vi "Read_Parameter_From_Data_Packet.vi"(8 "error in (no error)":errorcluster, 11 "Parameter name":string) -> (0 "error out":errorcluster, 3 "Parameter value out":string)   [LabVIEW 2017]
uses:
  Controls/Data Packets/Data_Packet_FGV_Commands.ctl
panel:
  out "Target test parameter value":string
  in  "Target test parameter":string
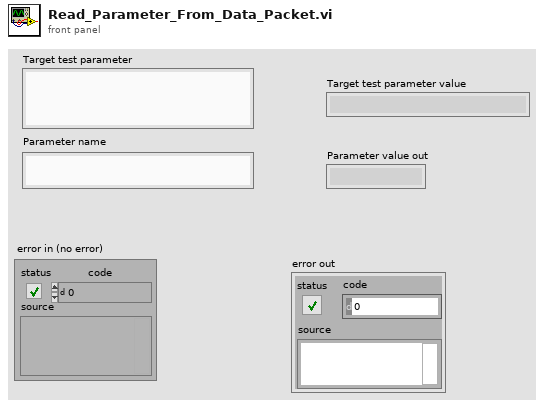
[diagram p1: front panel]
types:
  T1 = typedef "Data_Packet_FGV_Commands.ctl" = enum16{"Update all parameters from data packets", "Update Packet", "Load", "Read Packet Parameters", "Write Packet Parameters", "Read Packet Parameter", "Write Packet Parameter", "Read Data Packets", "Read Data Packet", "Read Data Packet by Parameter Name", "Get Parameter Node and Frame ID", "Read Data Packet from Node ID and Frame ID"}
  T2 = typedef "Data_Packet.ctl" = cluster{"Packet":T3, "Parameters":T7[], "Last Received Time (ms)":u64, "Receive count":i32, "Transmit count":i32, "Transmit interval (ms)":u32, "Last Transmitted Time (ms)":u64, "Receive interval (ms)":u32, "Transmit_Mode":T9, "Transmit Enable":bool, "Cyclic Transmit interval (ms)":u32}
  T3 = typedef "Packet.ctl" = cluster{"Raw Bytes":u8[], "Checksum":bool, "Direction":T4, "Processed Bytes":u8[], "Node ID":u8, "Packet type":T5, "Frame Data":u32, "Priority":T6, "Frame ID":u8}
  T4 = typedef "Packet_Direction.ctl" = enum16{"Transmit", "Receive", "Bidirectional"}
  T5 = typedef "Packet_Type.ctl" = enum16{"Data", "Connection Management", "Remote Request", "Error/Status"}
  T6 = typedef "Packet_Priority.ctl" = enum16{"LOW", "HIGH"}
  T7 = typedef "Parameter.ctl" = cluster{"Parameter name":string, "Node name":string, "Node ID":u8, "Frame name":string, "Frame ID":u8, "Data type":T8, "Start Bit":i32, "Bit Length":i32, "Factor":dbl, "Offset":dbl, "Minimum":dbl, "Maximum":dbl, "Descriptor":string, "Enum values":string[], "Value":string}
  T8 = typedef "Parameter_Data_Type.ctl" = enum16{"BOOL", "UNSIGNED", "SIGNED", "FLOAT32", "ENUM"}
  T9 = typedef "Data_Packet_Transmit_Mode.ctl" = enum16{"Disabled", "Single", "Cyclic"}
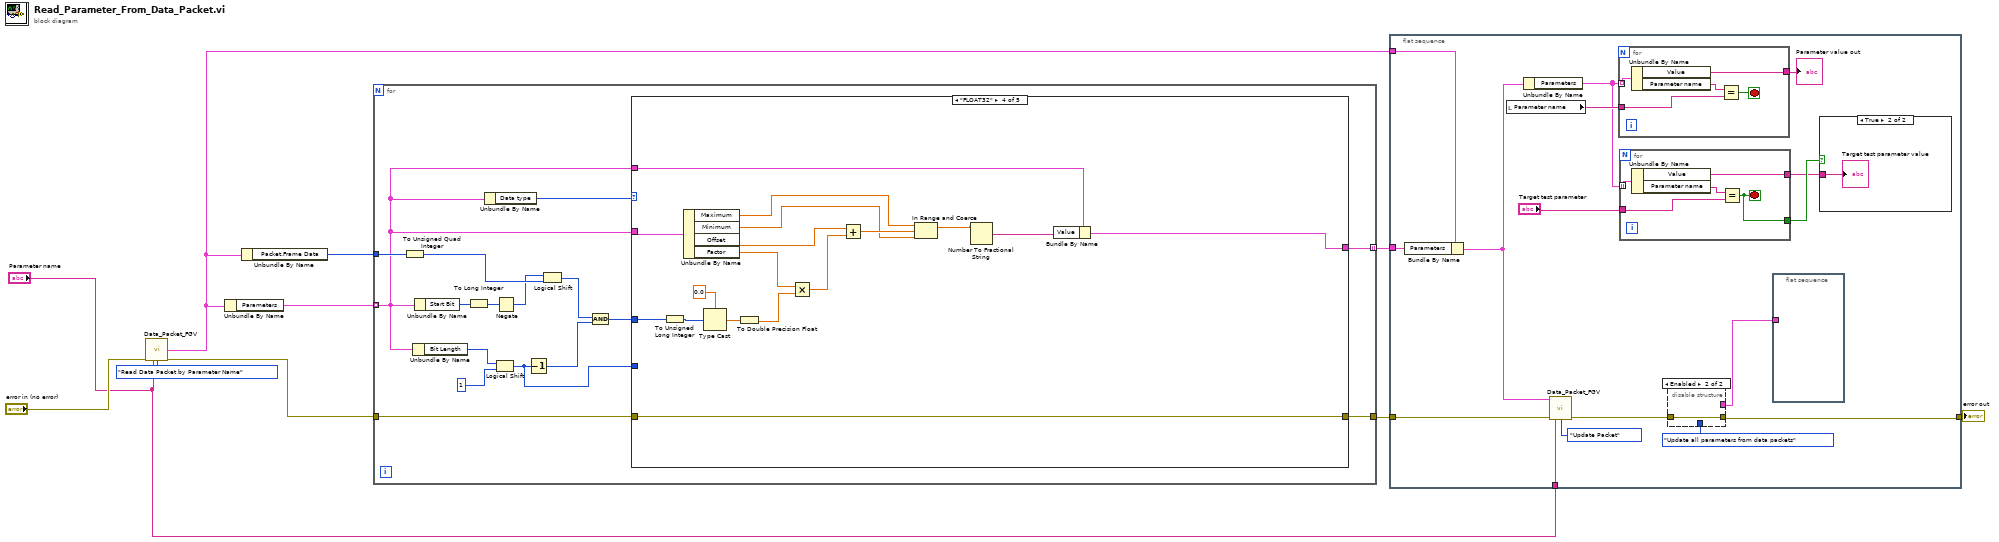
[diagram p0: block diagram]
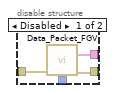
[diagram p2: hidden frame]
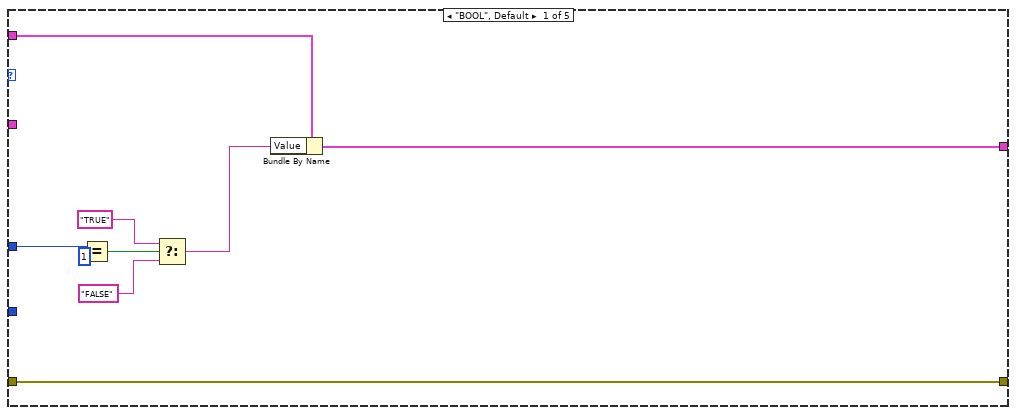
[diagram p4: hidden frame]
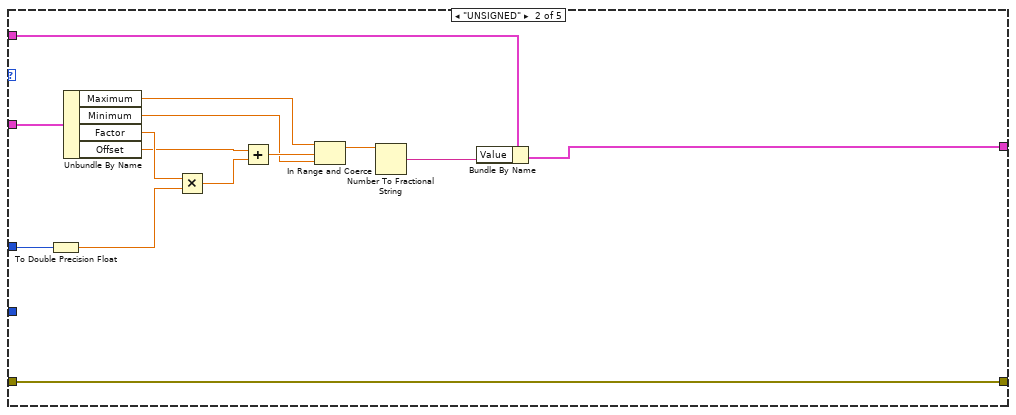
[diagram p5: hidden frame]
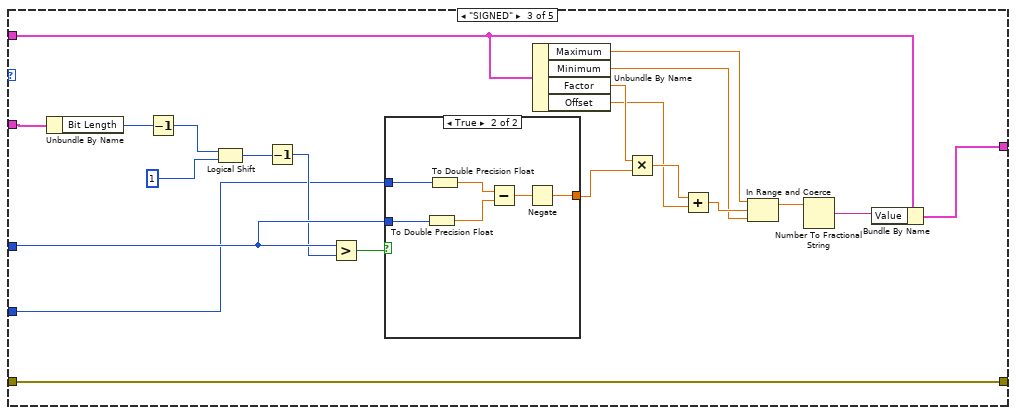
[diagram p6: hidden frame]
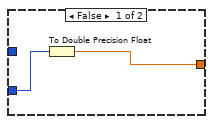
[diagram p7: hidden frame]
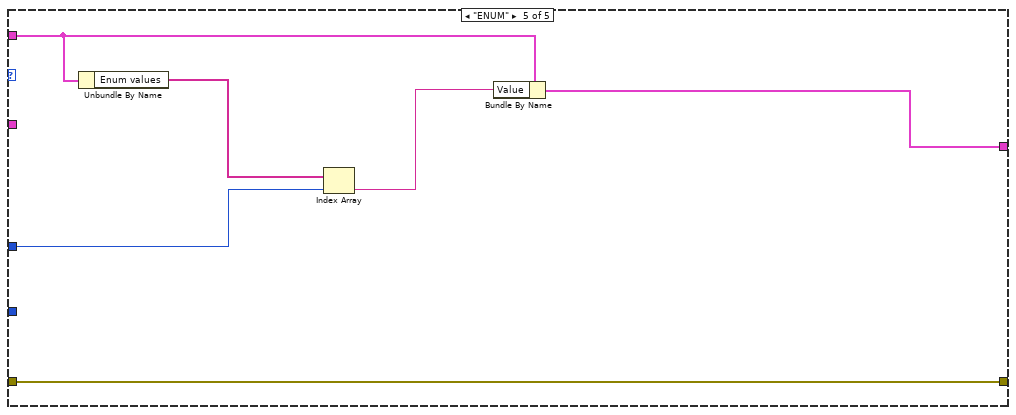
[diagram p8: hidden frame]
diagram:
  n1 = call "Data_Packet_FGV.vi"("error in (no error)"="error in (no error)", "Parameter name"="Parameter name", "Commands"=Data_Packet_FGV_Commands."Read Data Packet by Parameter Name") -> ("Data_Packet out"=w1:T2, "error out"=w7:errorcluster)  [unwired: 7 in, 4 out]
  n2 = Unbundle By Name(w1) -> ("Parameters"=w6:T7[])
  n3 = Unbundle By Name(w1) -> ("Packet.Frame Data"=w8:u32)
  n4 = for {
    tunnel: w8 -> [w26]
    tunnel: w7 -> [w15]
    tunnel: w6 -> [w13] mode=indexing
    tunnel: [w16] -> w3 mode=indexing
    tunnel: [w14] -> w5
    n5 = To Unsigned Quad Integer(1:w26) -> (0:w25:u64)
    n6 = Unbundle By Name(w13) -> ("Bit Length"=w20:i32)
    n7 = Unbundle By Name(w13) -> ("Start Bit"=w24:i32)
    n8 = To Long Integer(number=w24) -> (32bit integer=w23:i32)
    n9 = Unbundle By Name(w13) -> ("Data type"=w18:T8)
    n10 = Logical Shift(y=w20, x=u64 1) -> (x << y=w11:u64)
    n11 = Negate(x=w23) -> (-x=w22:i32)
    n12 = Decrement(x=w11) -> (x-1=w12:u64)
    n13 = Logical Shift(y=w22, x=w25) -> (x << y=w21:u64)
    n14 = And(x=w21, y=w12) -> (x .and. y?=w17:u64)
    n15 = case shown="\"FLOAT32\"" w18 {
      tunnel: w13 -> [w30 w40 w57 w82 w99]
      tunnel: w17 -> [w35 w49 w65 w95 w100]
      tunnel: [w28 w37 w55 w80 w97] -> w16
      tunnel: w15 -> [w27 w36 w59 w79 w96]
      tunnel: [w27 w36 w59 w79 w96] -> w14
      tunnel: w13 -> [_ w48 w70 w90 _]
      tunnel: w11 -> [_ _ w50 _ _]
      frame "BOOL", Default {
        n16 = Equal?(x=w35, y=u64 1) -> (x = y?=w33:bool)
        n17 = Select(t="TRUE", s=w33, f="FALSE") -> (s? t:f=w29:string)
        n18 = Bundle By Name(cluster=w30, "Value"=w29) -> (w28:T7)
      }
      frame "UNSIGNED" {
        n19 = To Double Precision Float(number=w49) -> (double precision float=w46:dbl)
        n20 = Unbundle By Name(w48) -> ("Maximum"=w42:dbl, "Minimum"=w41:dbl, "Factor"=w47:dbl, "Offset"=w45:dbl)
        n21 = Multiply(x=w47, y=w46) -> (x*y=w44:dbl)
        n22 = Add(x=w45, y=w44) -> (x+y=w43:dbl)
        n23 = In Range and Coerce(upper limit=w42, x=w43, lower limit=w41) -> (coerced(x)=w39:dbl)  [unwired: 1 out]
        n24 = Number To Fractional String(number=w39) -> (F-format string=w38:string)  [unwired: 3 in]
        n25 = Bundle By Name(cluster=w40, "Value"=w38) -> (w37:T7)
      }
      frame "SIGNED" {
        n26 = Unbundle By Name(w70) -> ("Bit Length"=w69:i32)
        n27 = Decrement(x=w69) -> (x-1=w68:i32)
        n28 = Logical Shift(y=w68, x=u64 1) -> (x << y=w66:u64)
        n29 = Decrement(x=w66) -> (x-1=w64:u64)
        n30 = Greater?(x=w65, y=w64) -> (0:w58:bool)
        n31 = case shown="True" w58 {
          tunnel: w65 -> [w71 w78]
          tunnel: [w72 w73] -> w62
          tunnel: w50 -> [_ w74]
          frame False {
            n32 = To Double Precision Float(number=w71) -> (double precision float=w72:dbl)
          }
          frame True {
            n33 = To Double Precision Float(number=w78) -> (double precision float=w76:dbl)
            n34 = To Double Precision Float(number=w74) -> (double precision float=w77:dbl)
            n35 = Subtract(x=w77, y=w76) -> (x-y=w75:dbl)
            n36 = Negate(x=w75) -> (-x=w73:dbl)
          }
        }
        n37 = Unbundle By Name(w57) -> ("Maximum"=w52:dbl, "Minimum"=w51:dbl, "Factor"=w63:dbl, "Offset"=w60:dbl)
        n38 = Multiply(x=w63, y=w62) -> (x*y=w61:dbl)
        n39 = Add(x=w61, y=w60) -> (x+y=w53:dbl)
        n40 = In Range and Coerce(upper limit=w52, x=w53, lower limit=w51) -> (coerced(x)=w54:dbl)  [unwired: 1 out]
        n41 = Number To Fractional String(number=w54) -> (F-format string=w56:string)  [unwired: 3 in]
        n42 = Bundle By Name(cluster=w57, "Value"=w56) -> (w55:T7)
      }
      frame "FLOAT32" {
        n43 = To Unsigned Long Integer(number=w95) -> (unsigned 32bit integer=w94:u32)
        n44 = Unbundle By Name(w90) -> ("Maximum"=w85:dbl, "Minimum"=w84:dbl, "Offset"=w88:dbl, "Factor"=w89:dbl)
        n45 = Type Cast(type=sgl 0.0 ("single precision float"), x=w94) -> (*(type *) &x=w92:sgl)
        n46 = To Double Precision Float(number=w92) -> (double precision float=w91:dbl)
        n47 = Multiply(x=w89, y=w91) -> (x*y=w87:dbl)
        n48 = Add(x=w88, y=w87) -> (x+y=w86:dbl)
        n49 = In Range and Coerce(upper limit=w85, x=w86, lower limit=w84) -> (coerced(x)=w83:dbl)  [unwired: 1 out]
        n50 = Number To Fractional String(number=w83) -> (F-format string=w81:string)  [unwired: 3 in]
        n51 = Bundle By Name(cluster=w82, "Value"=w81) -> (w80:T7)
      }
      frame "ENUM" {
        n52 = Unbundle By Name(w99) -> ("Enum values"=w101:string[])
        n53 = Index Array(array=w101, index=w100) -> (element=w98:string)
        n54 = Bundle By Name(cluster=w99, "Value"=w98) -> (w97:T7)
      }
    }
  }
  n55 = flat-sequence {
    tunnel: w5 -> [w117]
    tunnel: "Parameter name" -> [w116]
    tunnel: w3 -> [w114]
    tunnel: [w107] -> w2
    tunnel: w1 -> [w113]
    frame #0 {
      n56 = Bundle By Name(cluster=w113, "Parameters"=w114) -> (w110:T2)
      n57 = local read "Parameter name"() -> (w112:string)
      n58 = Unbundle By Name(w110) -> ("Parameters"=w105:T7[])
      n59 = call "Data_Packet_FGV.vi"("Data_Packet In"=w110, "error in (no error)"=w117, "Parameter name"=w116, "Commands"=Data_Packet_FGV_Commands."Update Packet") -> ("error out"=w109:errorcluster)  [unwired: 6 in, 5 out]
      n60 = for {
        tunnel: w105 -> [w133] mode=indexing
        tunnel: w112 -> [w131]
        tunnel: [w129] -> w111
        stop <- w130 stop-if-true
        n61 = Unbundle By Name(w133) -> ("Value"=w129:string, "Parameter name"=w132:string)
        n62 = Equal?(x=w132, y=w131) -> (x = y?=w130:bool)
      }
      "Parameter value out" <- w111
      n63 = for {
        tunnel: w105 -> [w128] mode=indexing
        tunnel: "Target test parameter" -> [w126]
        tunnel: [w125] -> w102
        tunnel: [w124] -> w103
        stop <- w124 stop-if-true
        n64 = Unbundle By Name(w128) -> ("Value"=w125:string, "Parameter name"=w127:string)
        n65 = Equal?(x=w127, y=w126) -> (x = y?=w124:bool)
      }
      n66 = disable-structure shown="Enabled" {
        disable-tunnel: w109 -> [w121 w122]
        disable-tunnel: Data_Packet_FGV_Commands."Update all parameters from data packets" ("Commands") -> [w120 _]
        disable-tunnel: [w119 w122] -> w107
        disable-tunnel: [w118 _] -> w106
        frame Disabled {
          n67 = call "Data_Packet_FGV.vi"("error in (no error)"=w121, "Commands"=w120) -> ("Parameters out"=w118:T7[], "error out"=w119:errorcluster)  [unwired: 8 in, 4 out]
        }
        frame Enabled {
        }
      }
      n68 = flat-sequence {
        tunnel: w106 -> [_]
        frame #0 {
        }
      }
      n69 = case shown="True" w103 {
        tunnel: w102 -> [_ w123]
        frame False {
        }
        frame True {
          "Target test parameter value" <- w123
        }
      }
    }
  }
  "error out" <- w2
